vi "Loop_SEN.vi"() -> ()   [LabVIEW 2017, in "Joystick.lvlib"]
uses:
  Joystick.lvlib
  <vilib>/Rock Robotics/WPI/Joystick/WPI_JoystickDeviceEnum.ctl
  Globals/Global_STOP.vi
  Global_Joystick Write_Data.vi
panel:
  out "POVs":i16[](array[numeric])
  out "Buttons":bool[](array[boolean])
  out "Axes":dbl[](array[numeric])
  out "Cycle Time (S)":dbl format="%.3g"
  in  "Target Time(ms)":u32=50
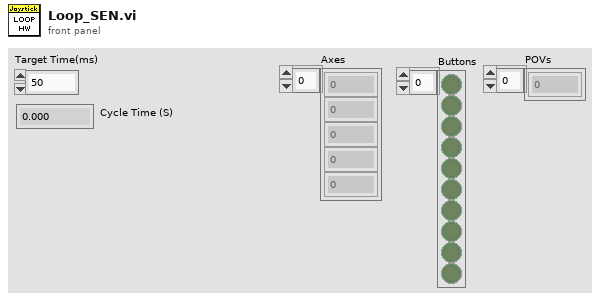
[diagram p1: front panel]
types:
  T1 = typedef "WPI_JoystickDeviceEnum.ctl" = enum16{"USB 0", "USB 1", "USB 2", "USB 3", "USB 4", "USB 5"}
  T2 = typedef "WPI_JoystickDevRef.ctl" = cluster{"Device":T1}
  T3 = cluster{"JoystickDevRef":T2, "Axes":dbl[], "Buttons":bool[], "POVs":i16[], "Target Time(ms)":u32, "Current Time":timestamp, "Previous Time":timestamp, "Cycle Time (S)":dbl}
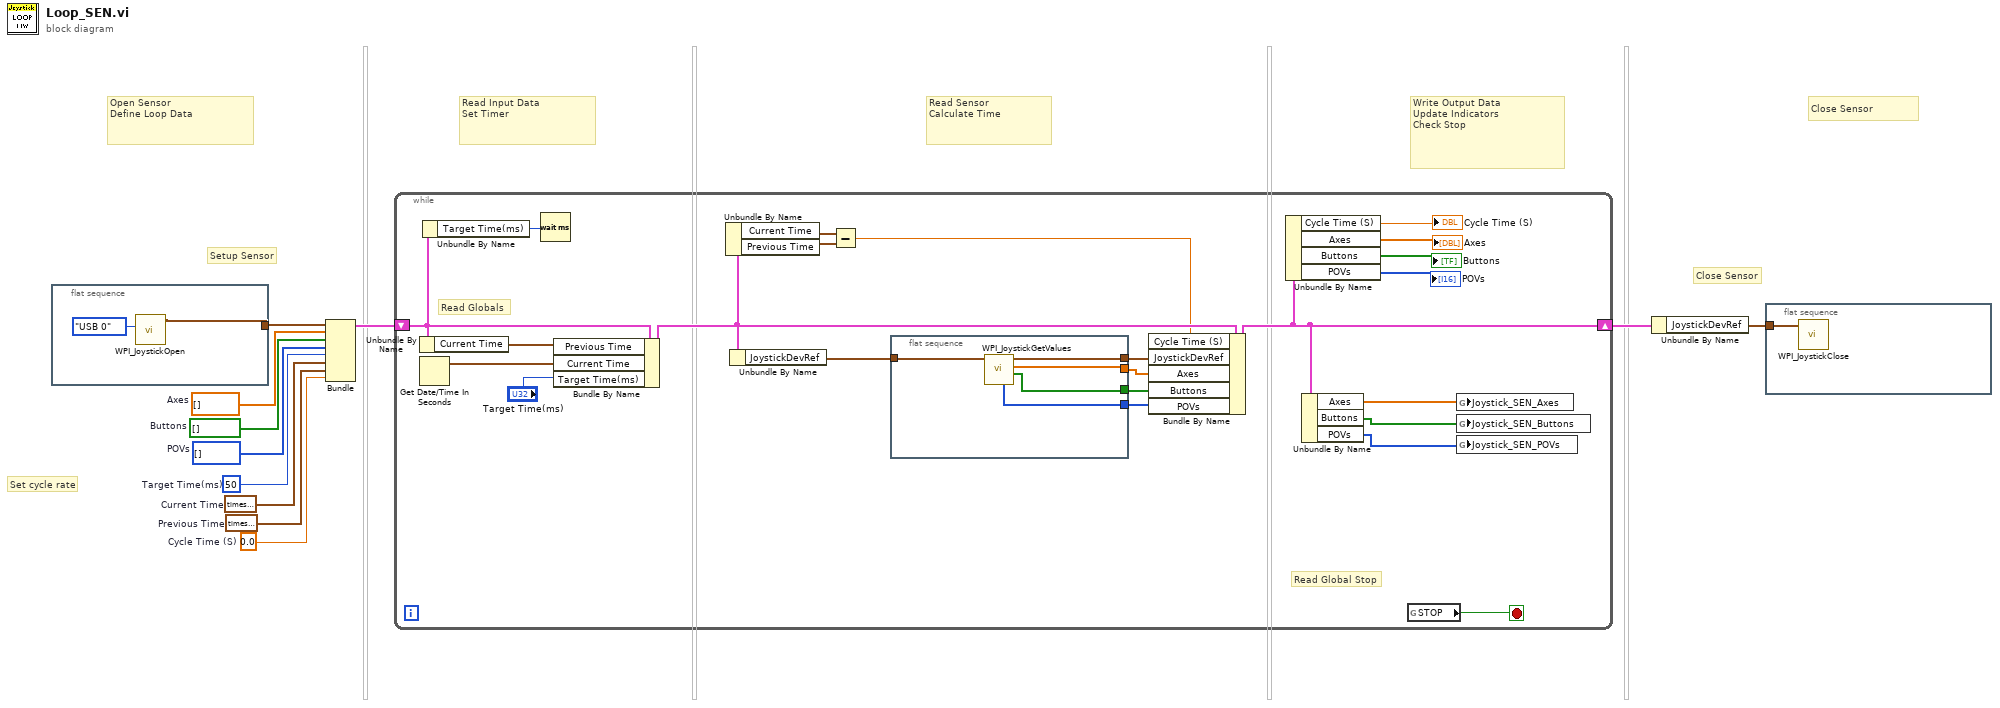
[diagram p0: block diagram]
diagram:
  w1 = i16[] []  # POVs
  w2 = bool[] []  # Buttons
  w3 = dbl[] []  # Axes
  w4 = 0.0  # Cycle Time (S)
  w11 = timestamp(0 s since 1904-01-01)  # Previous Time
  w10 = timestamp(0 s since 1904-01-01)  # Current Time
  w9 = u32 50  # Target Time(ms)
  # "Close Sensor"
  # "Write Output Data\nUpdate Indicators\nCheck Stop"
  # "Read Sensor\nCalculate Time"
  # "Read Input Data\nSet Timer"
  # "Open Sensor\nDefine Loop Data"
  # "Set cycle rate"
  # "Close Sensor"
  # "Setup Sensor"
  n1 = flat-sequence {
    tunnel: [w13] -> w6
    frame #0 {
      n2 = call <vilib>:"WPI_JoystickOpen.vi"("JoystickDevice"=WPI_JoystickDeviceEnum."USB 0") -> ("JoystickDevRef"=w13:T2)  [unwired: 10 in]
    }
  }
  n3 = Bundle("JoystickDevRef"=w6, "Axes"=w3, "Buttons"=w2, "POVs"=w1, "Target Time(ms)"=w9, "Current Time"=w10, "Previous Time"=w11, "Cycle Time (S)"=w4) -> (w7:T3)  [unwired: 1 in]
  n4 = while {
    shift-right: [w24] -> w5
    shift-left: w7 -> [w26]
    stop <- w36 stop-if-true
    # "Read Globals"
    # "Read Global Stop"
    n5 = Unbundle By Name(w26) -> ("Current Time"=w31:timestamp)
    n6 = Get Date/Time In Seconds() -> (seconds since 1Jan1904=w32:timestamp)
    n7 = Unbundle By Name(w26) -> ("Target Time(ms)"=w25:u32)
    n8 = Wait (ms)(milliseconds to wait=w25) -> ()  [unwired: 1 out]
    n9 = Bundle By Name(cluster=w26, "Previous Time"=w31, "Current Time"=w32, "Target Time(ms)"="Target Time(ms)") -> (w27:T3)
    n10 = Unbundle By Name(w27) -> ("Current Time"=w30:timestamp, "Previous Time"=w29:timestamp)
    n11 = Unbundle By Name(w27) -> ("JoystickDevRef"=w35:T2)
    n12 = Subtract(x=w30, y=w29) -> (x-y=w22:dbl)
    n13 = flat-sequence {
      tunnel: w35 -> [w41]
      tunnel: [w40] -> w34
      tunnel: [w39] -> w21
      tunnel: [w38] -> w20
      tunnel: [w37] -> w19
      frame #0 {
        n14 = call <vilib>:"WPI_JoystickGetValues.vi"("JoystickDevRef"=w41) -> ("Buttons"=w38:bool[], "Axes"=w39:dbl[], "JoystickDevRef"=w40:T2, "POVs"=w37:i16[])  [unwired: 6 in, 1 out]
      }
    }
    n15 = Bundle By Name(cluster=w27, "Cycle Time (S)"=w22, "JoystickDevRef"=w34, "Axes"=w21, "Buttons"=w20, "POVs"=w19) -> (w24:T3)
    n16 = Unbundle By Name(w24) -> ("Cycle Time (S)"=→"Cycle Time (S)":dbl, "Axes"=→"Axes":dbl[], "Buttons"=→"Buttons":bool[], "POVs"=→"POVs":i16[])
    n17 = Unbundle By Name(w24) -> ("Axes"=w33:dbl[], "Buttons"=w15:bool[], "POVs"=w14:i16[])
    n18 = global read "Global_STOP.vi" "STOP"() -> (w36:bool)
    n19 = global write "Global_Joystick Write_Data.vi" "Joystick_SEN_Axes"(w33) -> ()
    n20 = global write "Global_Joystick Write_Data.vi" "Joystick_SEN_Buttons"(w15) -> ()
    n21 = global write "Global_Joystick Write_Data.vi" "Joystick_SEN_POVs"(w14) -> ()
  }
  n22 = Unbundle By Name(w5) -> ("JoystickDevRef"=w8:T2)
  n23 = flat-sequence {
    tunnel: w8 -> [w42]
    frame #0 {
      n24 = call <vilib>:"WPI_JoystickClose.vi"("JoystickDevRef"=w42) -> ()  [unwired: 11 in]
    }
  }
